vi "IMAQ Padding.vi"(8 "error in (no error)":errorcluster, 10 "Final Size":i32=400, 11 "Image":T1) -> (0 "error out":errorcluster, 3 "Image Dst Out":T1)   [LabVIEW 2012, in "LightPipes.lvlib"]
uses:
  LightPipes.lvlib
  <vilib>/vision/Image Controls.llb/IMAQ Image.ctl
  <vilib>/vision/NI_Vision_Development_Module.lvlib
panel:
  out "Image":T1(plugin-control)
  out "cols padding":i32=5
  out "rows padding":i32=5
  # "Assuming Image is U16"
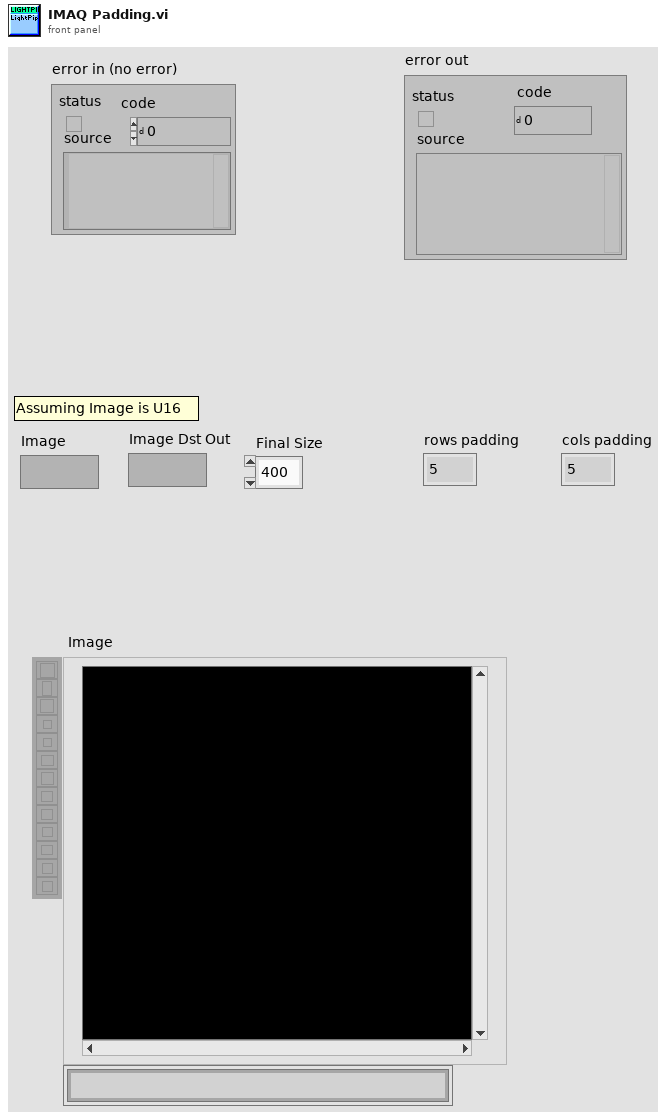
[diagram p1: front panel]
types:
  T1 = typedef "IMAQ Image.ctl" = refnum<image>
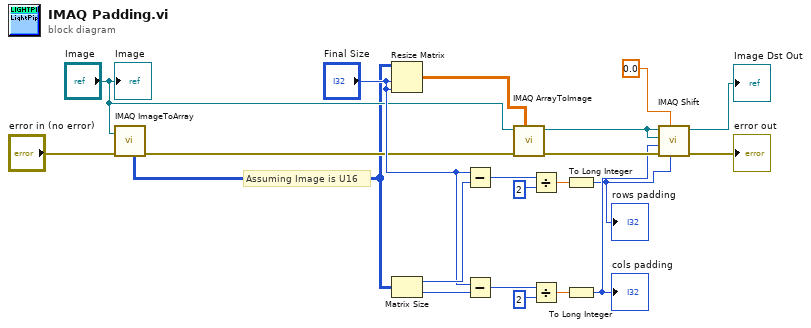
[diagram p0: block diagram]
diagram:
  # "Assuming Image is U16"
  n1 = call "IMAQ ImageToArray"("error in (no error)"="error in (no error)", "Image"="Image") -> ("Image Pixels (U16)"=w8:u16[][], "error out"=w11:errorcluster)  [unwired: 2 in, 3 out]
  n2 = Resize Matrix(1:"Final Size", 2:"Final Size", 4:w8) -> (0:w9:dbl[][])
  n3 = Matrix Size(0:w8) -> (1:w16:i32, 2:w15:i32)
  n4 = Subtract(x="Final Size", y=w16) -> (x-y=w21:i32)
  n5 = Subtract(x="Final Size", y=w15) -> (x-y=w19:i32)
  n6 = call "IMAQ ArrayToImage"("Image Pixels (U16)"=w9, "error in (no error)"=w11, "Image"="Image") -> ("error out"=w4:errorcluster, "Image Out"=w7:T1)  [unwired: 7 in]
  n7 = Divide(x=w21, y=2) -> (x/y=w13:dbl)
  n8 = Divide(x=w19, y=2) -> (x/y=w17:dbl)
  n9 = To Long Integer(number=w13) -> (32bit integer=w1:i32)
  "rows padding" <- w1
  n10 = To Long Integer(number=w17) -> (32bit integer=w2:i32)
  "cols padding" <- w2
  n11 = call "IMAQ Shift"("YOffset"=w1, "Replace Value"=sgl 0.0, "error in (no error)"=w4, "XOffset"=w2, "Image Dst"=w7, "Image Src"=w7) -> ("error out"=→"error out":errorcluster, "Image Dst Out"=→"Image Dst Out":T1)  [unwired: 4 in]
  "Image" <- "Image"
